vi "Boolean - No Error.vi"() -> ()   [LabVIEW 2017, in "Assertion.Tests.lvlib" / "Assert Is Boolean.lvlib"]
uses:
  Assert Is Boolean.lvlib
  Assertion/Assertion.lvlib
panel:
  out "error out":errorcluster
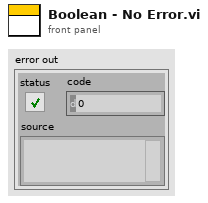
[diagram p1: front panel]
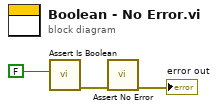
[diagram p0: block diagram]
diagram:
  n1 = call "Assert Is Boolean.vi"("Actual"=FALSE) -> ("error out"=w2:errorcluster)  [unwired: 10 in]
  n2 = call "Assert No Error.vi"("error in (no error)"=w2) -> ("error out"=→"error out":errorcluster)  [unwired: 10 in]
